vi "validated_timestamp_to_bool.vi"(1 "Cluster":T2) -> (0 "Cluster 2":T1)   [LabVIEW 2018]
uses:
  validated_u32.ctl
  validated_bool.ctl
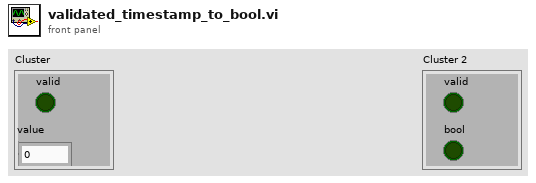
[diagram p1: front panel]
types:
  T1 = typedef "validated_bool.ctl" = cluster{"valid":bool, "bool":bool}
  T2 = typedef "validated_u32.ctl" = cluster{"valid":bool, "value":u32}
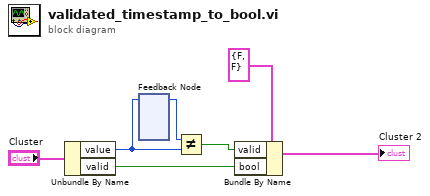
[diagram p0: block diagram]
diagram:
  n1 = Unbundle By Name("Cluster") -> ("value"=w6:u32, "valid"=w2:bool)
  n2 = feedback-in #1(w6) -> ()
  n3 = feedback #1() -> (w5:u32)  [unwired: 1 in]
  n4 = Not Equal?(x=w5, y=w6) -> (x != y?=w1:bool)
  n5 = Bundle By Name(cluster=T1 {"valid"=FALSE, "bool"=FALSE} ("Cluster 3"), "valid"=w1, "bool"=w2) -> (→"Cluster 2":T1)
